vi "unpack_calibration.vi"(10 "element_count":i32, 11 "calibration":u64) -> (2 "error":bool, 3 "calibration":sgl[](array[numeric]))   [LabVIEW 2023]
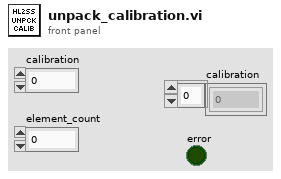
[diagram p1: front panel]
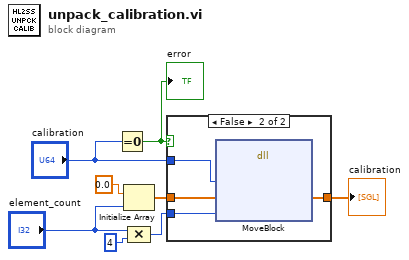
[diagram p0: block diagram]
diagram:
  n1 = Equal To 0?(x="calibration") -> (x = 0?=w5:bool)
  "error" <- w5
  n2 = Initialize Array(sgl 0.0 ("element"), "element_count") -> (w7:sgl[])
  n3 = Compound Arithmetic op=MULTIPLY("element_count", u64 4 ("dimension size")) -> (w6:u64)
  n4 = case shown="False" w5 {
    tunnel: w7 -> [w9 w11]
    tunnel: w6 -> [_ w10]
    tunnel: "calibration" -> [_ w13]
    tunnel: [w9 w12] -> w3
    frame True {
    }
    frame False {
      n5 = dll-call lib="LabVIEW" fn="MoveBlock"("ps"=w13, "pd"=w11, "size"=w10) -> ("pd"=w12:sgl[])  [unwired: 6 in, 2 out]
    }
  }
  "calibration" <- w3
